vi "Column DBL.vi"(8 "error in (no error)":errorcluster, 11 "SQL Statement in":refnum<class "SQL Statement.lvclass">) -> (0 "error out":errorcluster, 2 "DBL":dbl, 3 "SQL Statement out":refnum<class "SQL Statement.lvclass">)   [LabVIEW 2023, in "SQLite.lvlib" / "SQL Statement.lvclass"]
doc: "Returns the value in the next column as a LabVIEW DBL.\n\nNote: NULLs are extracted as NaN, rather than zero (as is normally done in SQLite3). Text and blobs also return NaN."
uses:
  SQL Statement.lvclass
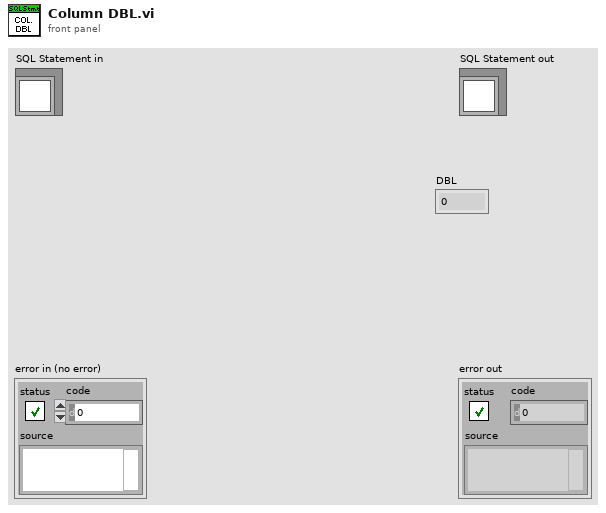
[diagram p1: front panel]
types:
  T1 = typedef "SQLite.lvlib/SQLITE Datatype.ctl" = enum32{"undefined type (0)", "SQLITE_INTEGER", "SQLITE_FLOAT", "SQLITE3_TEXT", "SQLITE_BLOB", "SQLITE_NULL", "undefined type"}
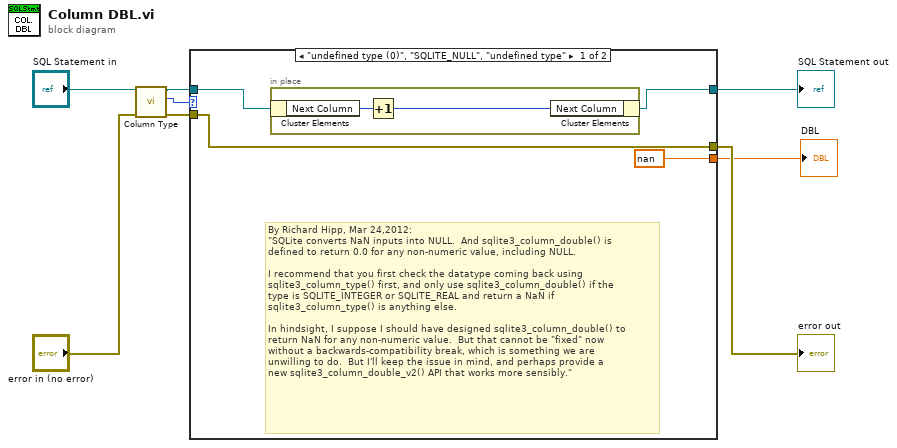
[diagram p0: block diagram]
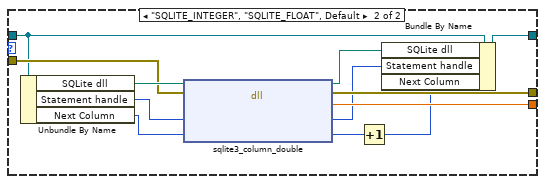
[diagram p2: hidden frame]
diagram:
  n1 = call "Column Type.vi"("error in (no error)"="error in (no error)", "SQL Statement in"="SQL Statement in") -> ("error out"=w3:errorcluster, "SQLite3 type"=w2:T1, "SQL Statement out"=w4:refnum<class "SQL Statement.lvclass">)  [unwired: 7 in]
  n2 = case shown="\"undefined type (0)\", \"SQLITE_NULL\", \"undefined type\"" w2 {
    tunnel: [w12 w24] -> w7
    tunnel: [nan ("DBL") w23] -> w5
    tunnel: w4 -> [w10 w20]
    tunnel: w3 -> [w12 w21]
    tunnel: [w9 w19] -> w1
    frame "undefined type (0)", "SQLITE_NULL", "undefined type" {
      # "By Richard Hipp, Mar 24,2012:\n\"SQLite converts NaN inputs into NULL.  And sqlite3_column_double() is\ndefined to return 0.0 for any non-numeric value, including NULL.\n\nI recommend that you first check the datatype coming back using\nsqlite3_column_type() first, and only use sqlite3_column_double() if the\ntype is SQLITE_INTEGER or SQLITE_REAL and return a NaN if\nsqlite3_column_type() is anything else.\n\nIn hindsight, I suppose I should have designed sqlite3_column_double() to\nreturn NaN for any non-numeric value.  But that cannot be \"fixed\" now\nwithout a backwards-compatibility break, which is something we are\nunwilling to do.  But I'll keep the issue in mind, and perhaps provide a\nnew sqlite3_column_double_v2() API that works more sensibly.\""
      n3 = in-place {
        n4 = in-place-cluster #1(w10) -> ("Next Column"=w14:i32)
        n5 = Increment(x=w14) -> (x+1=w13:i32)
        n6 = in-place-cluster #1("Next Column"=w13) -> (w9:refnum<class "SQL Statement.lvclass">)
      }
    }
    frame "SQLITE_INTEGER", "SQLITE_FLOAT", Default {
      n7 = Unbundle By Name(w20) -> ("SQLite dll"=w26:path, "Statement handle"=w25:u64, "Next Column"=w22:i32)
      n8 = dll-call lib="C:/LabVIEW_JDP/Support/SQLite/sqlite3.dll" fn="sqlite3_column_double"(path in=w26, error in=w21, "Statement"=w25, "Column"=w22) -> (path out=w18:path, error out=w24:errorcluster, "DBL"=w23:dbl, "Statement"=w17:u64, "Column"=w16:i32)  [unwired: 1 in]
      n9 = Increment(x=w16) -> (x+1=w15:i32)
      n10 = Bundle By Name(cluster=w20, "SQLite dll"=w18, "Statement handle"=w17, "Next Column"=w15) -> (w19:refnum<class "SQL Statement.lvclass">)
    }
  }
  "error out" <- w7
  "SQL Statement out" <- w1
  "DBL" <- w5
